vi "CheckCondition.vi"(8 "Negate":bool, 10 "Condition":i32) -> (2 "Condition True?":bool)   [LabVIEW 2013]
uses:
  Robot Global Data.vi
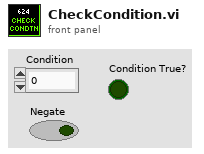
[diagram p1: front panel]
types:
  T1 = typedef "Dashboard UDP Packet.ctl" = cluster{"Camera":T2, "Gyro":T3, "Encoder":T5, "Auto Shift":T6, "Auton":T7, "Drive/Ramp X":dbl, "Drive/Ramp Y":dbl, "Drive/Battery Cutoff":dbl, "Pressure/Compressor Min Voltage":dbl, "Pressure/Compressor Delay":dbl, "Controller/Strafe Correction":bool, "Shooter":T8, "Rollers":T9, "Abort":bool, "Finish":bool, "IR Halo Sustain Time":dbl, "Disable Compressor":bool, "Center Omni Drive Delay":i32, "Vision Mode":T10, "Radius Throttle":bool, "Fieldcentric":T11, "Roll":T12, "Stick Deadband":dbl}
  T2 = typedef "Camera Controls.ctl" = cluster{"Camera/View Angle X":dbl, "Camera/Goal Track Timeout":dbl, "Camera/View Angle Y":dbl, "Camera/Goal Exposure":dbl, "Camera/Vision Receive Timeout":dbl, "Camera/Offset 1":dbl, "Camera/Offset 2":dbl}
  T3 = typedef "Gyro Controls.ctl" = cluster{"Gyro/Angle Tolerance":dbl, "Gyro/Steer Closeness Threshold":dbl, "Steer PID":T4, "Steer Close PID":T4}
  T4 = typedef "PID Params.ctl" = cluster{"max":dbl, "min":dbl, "P":dbl, "I":dbl, "D":dbl}
  T5 = typedef "Encoder Controls.ctl" = cluster{"Encoders/Reset":bool, "Encoders/Omni Constant":dbl, "Encoders/Omni Tick Constant":dbl, "Encoders/Left Constant":dbl, "Encoders/Right Constant":dbl, "Encoders/Right Tick Constant":dbl}
  T6 = typedef "Auto Shift Controls.ctl" = cluster{"AutoShift/Upshift Throttle Accel":dbl, "AutoShift/Speed Threshold":dbl, "AutoShift/Upshift Throttle":dbl, "AutoShift/Upshift Accel":dbl, "AutoShift/Downshift Accel":dbl, "AutoShift/Downshift Throttle":dbl, "AutoShift/Delay":dbl, "AutoShift/Enabled":bool}
  T7 = typedef "Auton Controls.ctl" = cluster{"Auton/Left Shoot X-Coord":dbl, "Auton/Right Shoot X-Coord":dbl, "DistDrive/Distance Stop Threshold":dbl, "DistDrive/Max Stop Speed":dbl, "Auton/Back Piston Time":dbl, "Auton/Manual Hot":bool, "Auton/Manual Hot Right":bool, "Default X PID":T4, "Default Y PID":T4, "Half Over Delay":dbl}
  T8 = typedef "Shooter Controls.ctl" = cluster{"Shooter/Reset Time":dbl, "Shooter/Release Delay":dbl, "Shooter/Pressure Steady Time":dbl, "Shooter/Misfire Delay":dbl, "Shooter/Ball Settle Time":dbl, "Shooter/Line IR Delay":dbl, "Pressure/Upper PSI Time":dbl, "Pressure/Lower PSI Time":dbl, "Shooter/Punch Delay":dbl, "Shooter/Target Pressure":dbl, "Pressure/Line B":dbl, "Pressure/Line M":dbl, "Pressure/Shooter M":dbl, "Pressure/Shooter B":dbl, "Halo Time":dbl, "Soft Release Delay":dbl, "Soft Unpin Delay":dbl, "Soft Shoot Delay":dbl}
  T9 = typedef "Roller Controls.ctl" = cluster{"Roller/Load IRs Verify Time":dbl, "Roller/Center IR Latch Time":dbl, "Roller/Speed Front":dbl, "Roller/Speed Back":dbl, "Roller/Entry Timeout":dbl, "Roller/To Center Timeout":dbl, "Roller/Sustain Time":dbl, "Roller/Verify Center Time":dbl}
  T10 = typedef "Vision Mode.ctl" = enum16{"Normal", "Extreme Left", "Extreme Right"}
  T11 = typedef "Fieldcentric Controls.ctl" = cluster{"Relative Angle":bool, "Point Robot":bool, "X/Y ratio low":dbl, "Steering Gain":dbl, "Force Omni Down":bool, "Enable":bool, "X/Y ratio high":dbl}
  T12 = typedef "Roll Maneuver.ctl" = cluster{"X 1":dbl, "Y 1":dbl, "Y 2":dbl, "X 2":dbl, "Y 3":dbl, "X 3":dbl, "Time 1":i32, "Time 2":i32, "Time 3":i32, "Angle Start":dbl, "Angle End":dbl, "Angle Linearity":dbl}
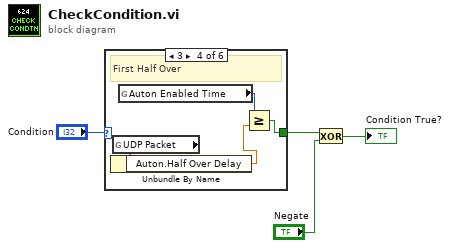
[diagram p0: block diagram]
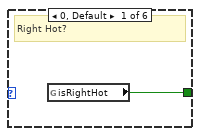
[diagram p2: hidden frame]
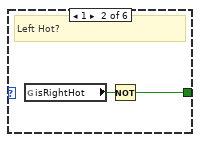
[diagram p3: hidden frame]
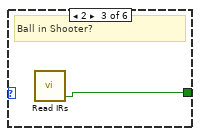
[diagram p4: hidden frame]
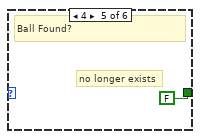
[diagram p5: hidden frame]
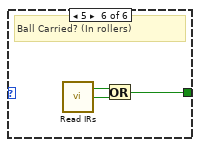
[diagram p6: hidden frame]
diagram:
  n1 = case shown="3" "Condition" {
    tunnel: [w5 w6 w8 w11 FALSE ("Center") w14] -> w3
    frame 0, Default {
      # "Right Hot?"
      n2 = global read "Robot Global Data.vi" "isRightHot"() -> (w5:bool)
    }
    frame 1 {
      # "Left Hot?"
      n3 = global read "Robot Global Data.vi" "isRightHot"() -> (w7:bool)
      n4 = Not(x=w7) -> (.not. x?=w6:bool)
    }
    frame 2 {
      # "Ball in Shooter?"
      n5 = call "Read IRs.vi"() -> ("Center"=w8:bool)  [unwired: 2 in, 3 out]
    }
    frame 3 {
      # "First Half Over"
      n6 = global read "Robot Global Data.vi" "UDP Packet"() -> (w10:T1)
      n7 = Unbundle By Name(w10) -> ("Auton.Half Over Delay"=w9:dbl)
      n8 = global read "Robot Global Data.vi" "Auton Enabled Time"() -> (w12:u32)
      n9 = Greater Or Equal?(x=w12, y=w9) -> (x >= y?=w11:bool)
    }
    frame 4 {
      # "no longer exists"
      # "Ball Found?"
    }
    frame 5 {
      # "Ball Carried? (In rollers)"
      n10 = call "Read IRs.vi"() -> ("Back"=w15:bool, "Front"=w16:bool)  [unwired: 2 in, 2 out]
      n11 = Or(x=w16, y=w15) -> (x .or. y?=w14:bool)
    }
  }
  n12 = Exclusive Or(1:"Negate", 2:w3) -> (0:→"Condition True?":bool)
